vi "Dequeue Message.vi"(8 "error in (no error)":cluster{"状态":bool, "代码":i32, "源":string} caption="错误输入（无错误）", 11 "消息队列":refnum<queue>) -> (0 "error out":cluster{"状态":bool, "代码":i32, "源":string} caption="错误输出", 1 "消息数据":variant, 2 "消息":string, 3 "消息队列副本":refnum<queue>)   [LabVIEW 2022 SP3, in "Message Queue.lvlib"]
doc: "本VI从消息队列中取出消息。"
uses:
  Message Queue.lvlib
  Message Cluster.ctl
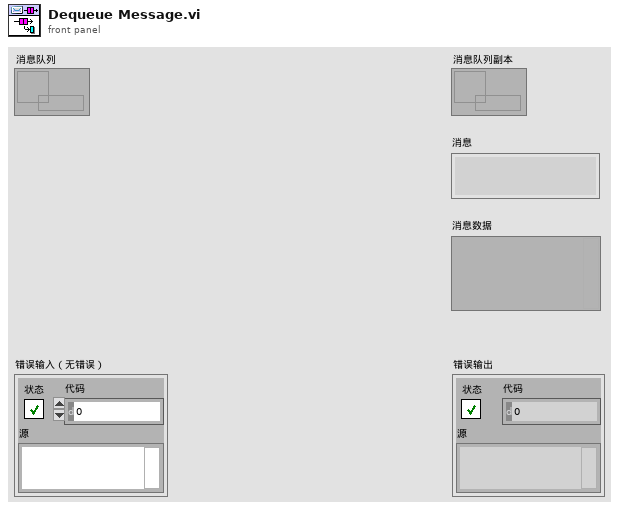
[diagram p1: front panel]
types:
  T1 = typedef "Message Queue.lvlib/Message Cluster.ctl" = cluster{"消息":string, "消息数据":variant}
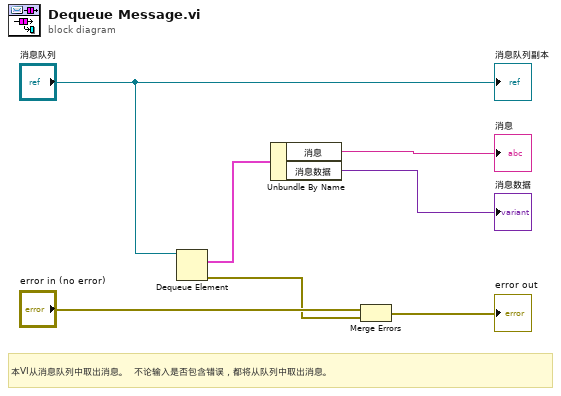
[diagram p0: block diagram]
diagram:
  # "本VI从消息队列中取出消息。  不论输入是否包含错误，都将从队列中取出消息。"
  n1 = Dequeue Element(queue="消息队列") -> (element=w4:T1, error out=w1:errorcluster)  [unwired: 2 in, 2 out]
  n2 = Unbundle By Name(w4) -> ("消息"=→"消息":string, "消息数据"=→"消息数据":variant)
  n3 = Merge Errors("error in (no error)", w1) -> (→"error out":errorcluster)
  "消息队列副本" <- "消息队列"
